vi "Shooter.vi"   [LabVIEW 2013]
uses:
  <vilib>/Rock Robotics/WPI/Solenoid/WPI_SolenoidValue.ctl
  <vilib>/Rock Robotics/WPI/Solenoid/WPI_SolenoidSetEnum.vi
  Robot Global Data.vi
types:
  T1 = typedef "WPI_SolenoidValue.ctl" = enum16{"Off", "On", "Forward", "Reverse"}
  T2 = typedef "WPI_SolenoidDevRef.ctl" = cluster{"DevStatus":errorcluster, "Solenoid Module":T3, "Forward Solenoid Channel":T4, "Reverse Solenoid Channel":T4}
  T3 = typedef "FPGA_TypedefSolenoidModule.ctl" = enum16{"Solenoid Module 1", "Solenoid Module 2"}
  T4 = typedef "WPI_SolenoidChannel.ctl" = enum8{"Solenoid 1", "Solenoid 2", "Solenoid 3", "Solenoid 4", "Solenoid 5", "Solenoid 6", "Solenoid 7", "Solenoid 8", "Invalid"}
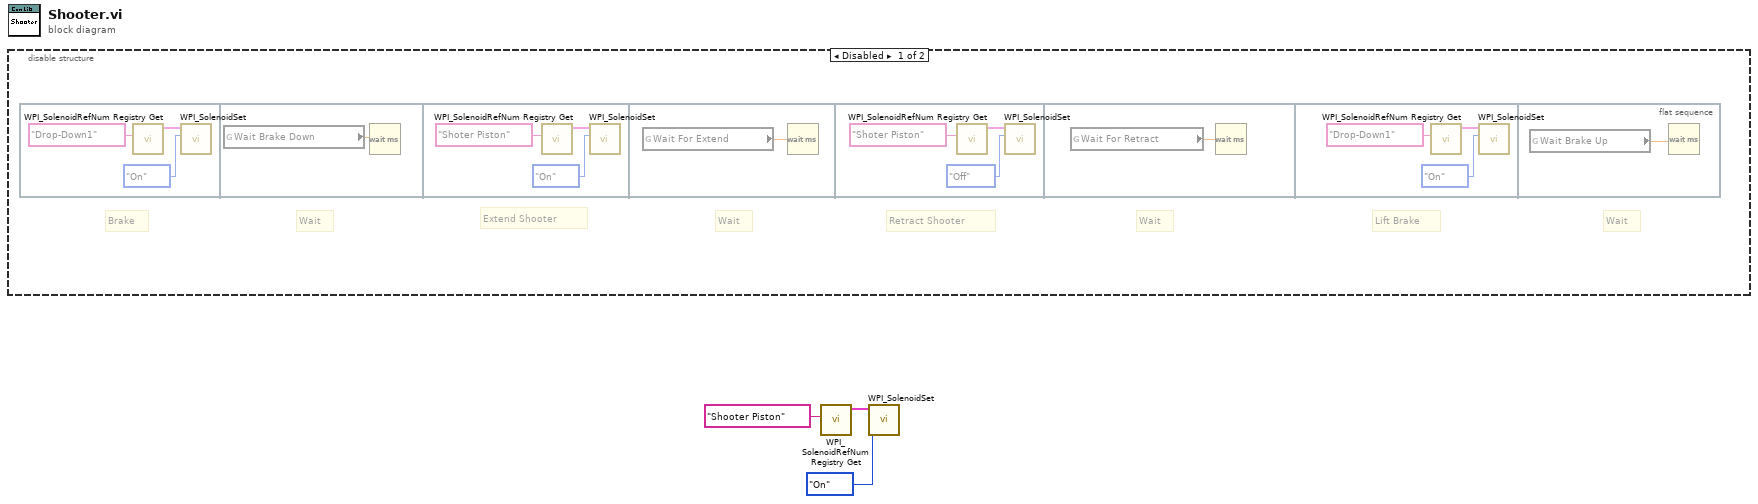
[diagram p0: block diagram]
diagram:
  n1 = disable-structure shown="Disabled" {
    frame Disabled {
      # "Wait"
      # "Lift Brake"
      # "Wait"
      # "Retract Shooter"
      # "Wait"
      # "Extend Shooter"
      # "Wait"
      # "Brake"
      n2 = flat-sequence {
        frame #0 {
          n3 = call <vilib>:"WPI_SolenoidRefNum Registry Get.vi"("refnum name"="Drop-Down1") -> ("SolenoidDevRef"=w5:T2)  [unwired: 9 in, 1 out]
          n4 = call-poly <vilib>:"WPI_SolenoidSet.vi"("Value"=WPI_SolenoidValue."On", "SolenoidDevRef"=w5) -> ()  [unwired: 8 in, 2 out]
        }
        frame #1 {
          n5 = global read "Robot Global Data.vi" "Wait Brake Down"() -> (w7:dbl)
          n6 = Wait (ms)(milliseconds to wait=w7) -> ()  [unwired: 1 out]
        }
        frame #2 {
          n7 = call <vilib>:"WPI_SolenoidRefNum Registry Get.vi"("refnum name"="Shoter Piston") -> ("SolenoidDevRef"=w8:T2)  [unwired: 9 in, 1 out]
          n8 = call-poly <vilib>:"WPI_SolenoidSet.vi"("Value"=WPI_SolenoidValue."On", "SolenoidDevRef"=w8) -> ()  [unwired: 8 in, 2 out]
        }
        frame #3 {
          n9 = global read "Robot Global Data.vi" "Wait For Extend"() -> (w11:dbl)
          n10 = Wait (ms)(milliseconds to wait=w11) -> ()  [unwired: 1 out]
        }
        frame #4 {
          n11 = call <vilib>:"WPI_SolenoidRefNum Registry Get.vi"("refnum name"="Shoter Piston") -> ("SolenoidDevRef"=w14:T2)  [unwired: 9 in, 1 out]
          n12 = call-poly <vilib>:"WPI_SolenoidSet.vi"("Value"=WPI_SolenoidValue."Off", "SolenoidDevRef"=w14) -> ()  [unwired: 8 in, 2 out]
        }
        frame #5 {
          n13 = global read "Robot Global Data.vi" "Wait For Retract"() -> (w15:dbl)
          n14 = Wait (ms)(milliseconds to wait=w15) -> ()  [unwired: 1 out]
        }
        frame #6 {
          n15 = call <vilib>:"WPI_SolenoidRefNum Registry Get.vi"("refnum name"="Drop-Down1") -> ("SolenoidDevRef"=w17:T2)  [unwired: 9 in, 1 out]
          n16 = call-poly <vilib>:"WPI_SolenoidSet.vi"("Value"=WPI_SolenoidValue."On", "SolenoidDevRef"=w17) -> ()  [unwired: 8 in, 2 out]
        }
        frame #7 {
          n17 = global read "Robot Global Data.vi" "Wait Brake Up"() -> (w19:dbl)
          n18 = Wait (ms)(milliseconds to wait=w19) -> ()  [unwired: 1 out]
        }
      }
    }
    frame Enabled {
    }
  }
  n19 = call <vilib>:"WPI_SolenoidRefNum Registry Get.vi"("refnum name"="Shooter Piston") -> ("SolenoidDevRef"=w2:T2)  [unwired: 9 in, 1 out]
  n20 = call-poly <vilib>:"WPI_SolenoidSet.vi"("Value"=WPI_SolenoidValue."On", "SolenoidDevRef"=w2) -> ()  [unwired: 8 in, 2 out]
